vi "Close Configuration Resource.vi"(8 "error in (no error)":errorcluster, 11 "TransientConfiguration in":refnum<class "TransientConfiguration.lvclass">) -> (0 "error out":errorcluster, 3 "TransientConfiguration out":refnum<class "TransientConfiguration.lvclass">)   [LabVIEW 2019, in "TransientConfiguration.lvclass"]
uses:
  <vilib>/gpm_packages/@cs/Configuration/Source/TransientConfiguration/TransientConfiguration.lvclass
  <vilib>/gpm_packages/@cs/Configuration/Source/TransientConfiguration/TransientConfiguration.lvclass/TransientConfiguration.ctl
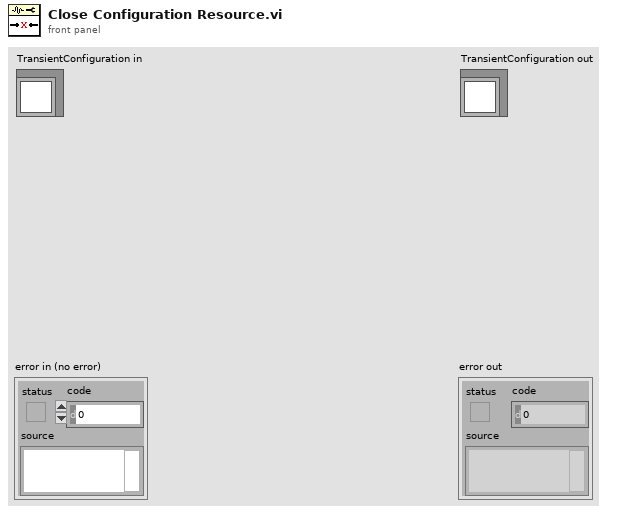
[diagram p1: front panel]
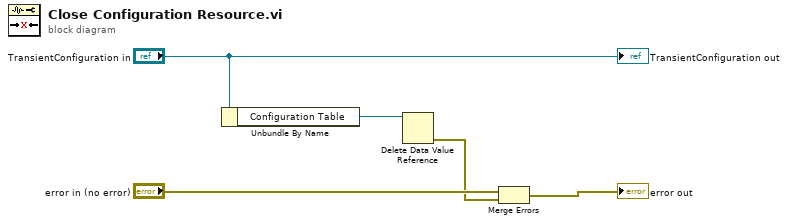
[diagram p0: block diagram]
diagram:
  n1 = Unbundle By Name("TransientConfiguration in") -> ("Configuration Table"=w3:refnum<data-value>)
  n2 = Delete Data Value Reference(data value reference=w3) -> (error out=w1:errorcluster)  [unwired: 1 in, 1 out]
  n3 = Merge Errors("error in (no error)", w1) -> (→"error out":errorcluster)
  "TransientConfiguration out" <- "TransientConfiguration in"
